vi "Process Mouse Up.vi"(0 "FSM.Graph in":T2, 5 "Display State In":T3, 7 "Coords":T4, 9 "PlatMods":T1, 11 "Editor Ref":refnum<vi>) -> (4 "FSM.Graph out":T2, 6 "Display State Out":T3, 10 "Refresh":bool)   [LabVIEW 2015, in "FSM Editor.xctl"]
uses:
  FSM Editor.xctl
  <vilib>/Utility/miscctls.llb/LVPoint32TypeDef.ctl
  State.vi
  Classes/FSM.Port/FSM.Port.lvclass
  Drag Mode.ctl
  Events.ctl
  NodeAdded.ctl
  NodeSelected.ctl
  EdgeEventData.ctl
  Data.vi
  Classes/FSM.Graph/FSM.Graph.lvclass
  Classes/FSM.Port/FSM.Port.lvclass/FSM.Port.ctl
  Classes/FSM.Graph/FSM.Graph.lvclass/FSM.Graph.ctl
  Classes/FSM.Port/Read belongsTo.vi
  Classes/FSM.Graph/Read selectedNodes.vi
  Classes/FSM.Graph/Read selectedEdge.vi
  Classes/FSM.Graph/Write selectedEdge.vi
  <vilib>/Utility/cursorutil.llb/Set Cursor (Icon Pict).vi
  Classes/FSM.Edge/FSM.Edge.lvclass
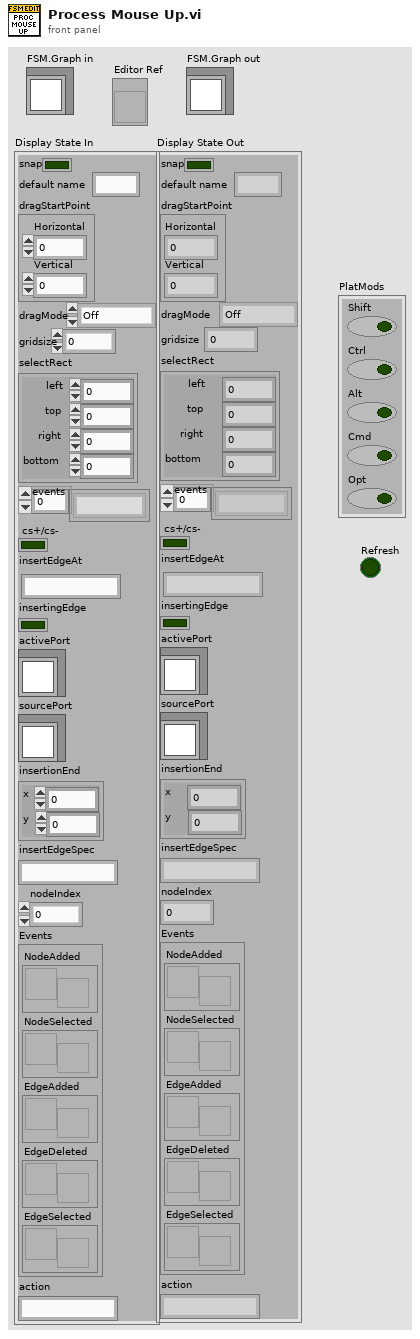
[diagram p1: front panel]
types:
  T1 = cluster{"Shift":bool, "Ctrl":bool, "Alt":bool, "Cmd":bool, "Opt":bool}
  T2 = typedef "FSM Editor.xctl/Data.vi" = refnum<class "FSM.Graph.lvclass">
  T3 = typedef "FSM Editor.xctl/State.vi" = cluster{"snap":bool, "default name":string, "dragStartPoint":T4, "dragMode":T5, "gridsize":dbl, "selectRect":cluster{"left":i16, "top":i16, "right":i16, "bottom":i16}, "events":string[], "cs+/cs-":bool, "insertEdgeAt":string, "insertingEdge":bool, "activePort":refnum<class "FSM.Port.lvclass">, "sourcePort":refnum<class "FSM.Port.lvclass">, "insertionEnd":cluster{"x":i16, "y":i16}, "insertEdgeSpec":string, "nodeIndex":i32, "Events":T6, "action":string}
  T4 = typedef "LVPoint32TypeDef.ctl" = cluster{"Horizontal":i32, "Vertical":i32}
  T5 = typedef "Drag Mode.ctl" = enum16{"Off", "NodePending", "Nodes", "Pan", "Select", "EdgeInsertion", "EdgePoint", "EdgeLabel"}
  T6 = typedef "FSM Editor.xctl/Events.ctl" = cluster{"NodeAdded":refnum<user-event>, "NodeSelected":refnum<user-event>, "EdgeAdded":refnum<user-event>, "EdgeDeleted":refnum<user-event>, "EdgeSelected":refnum<user-event>}
  T7 = enum16{"Off", "NodePending", "Nodes", "Pan", "Select", "EdgeInsertion", "EdgePoint", "Edgelabel"}
  T8 = cluster{"SourceName":string, "TargetName":string, "Accessors:Text":string, "Type":string}
  T9 = cluster{"left":i16, "top":i16, "right":i16, "bottom":i16}
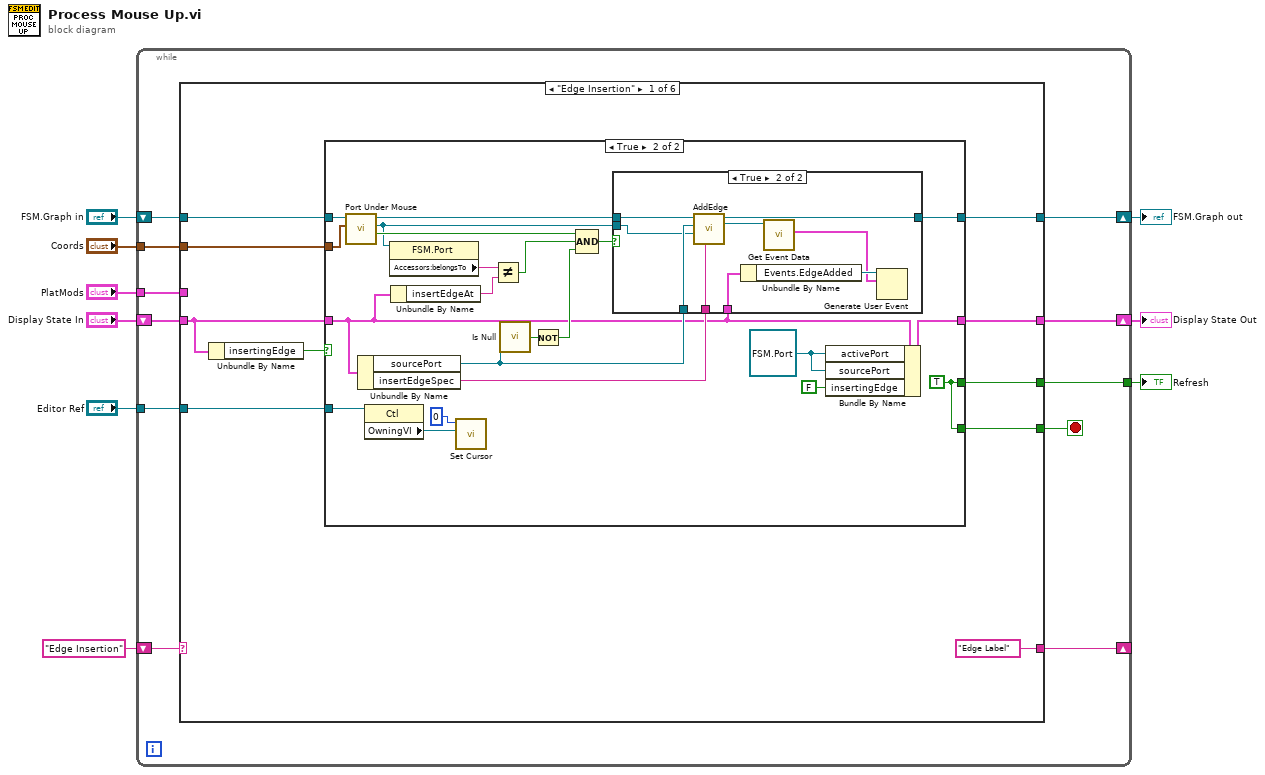
[diagram p0: block diagram]
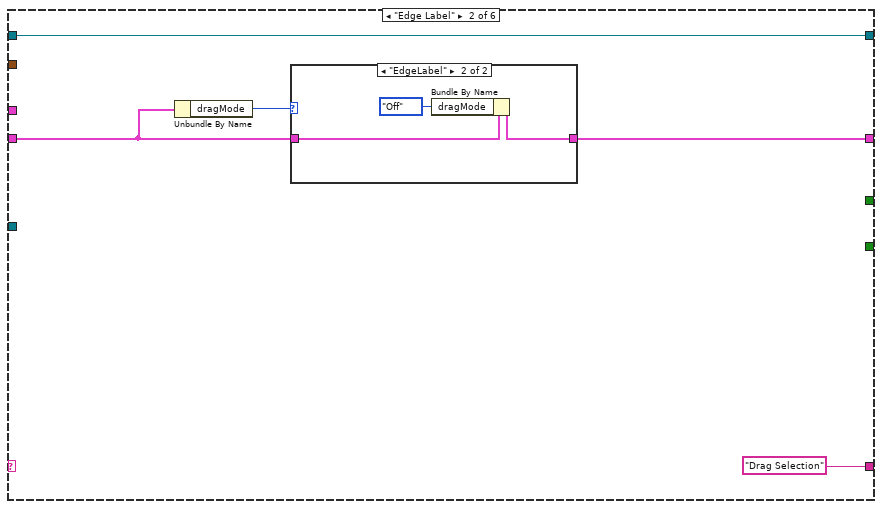
[diagram p4: hidden frame]
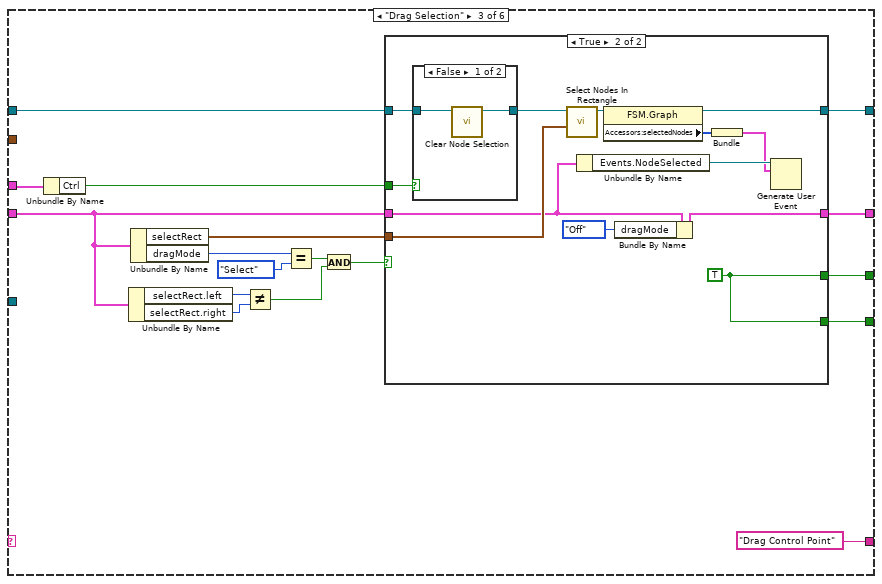
[diagram p6: hidden frame]
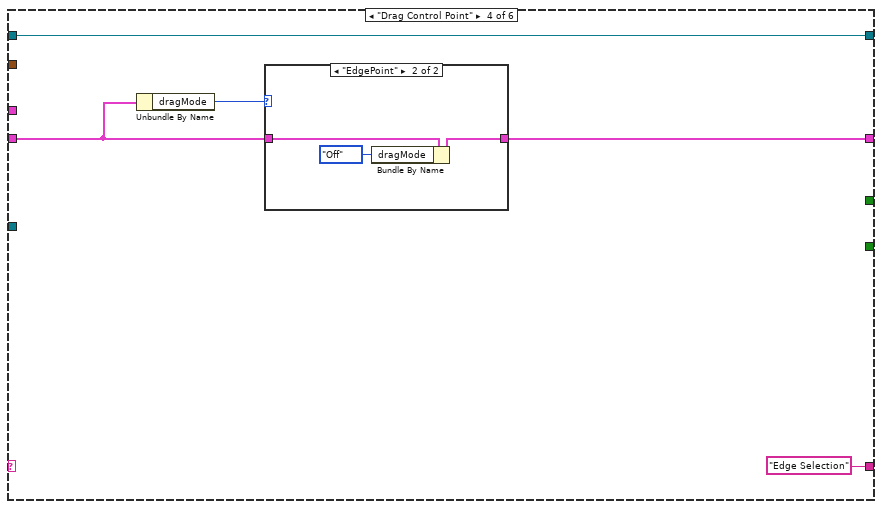
[diagram p9: hidden frame]
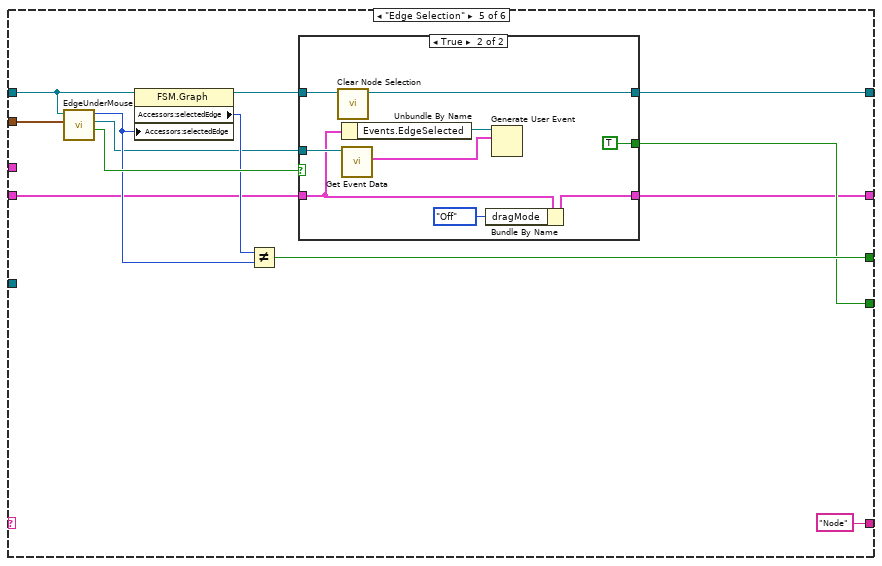
[diagram p11: hidden frame]
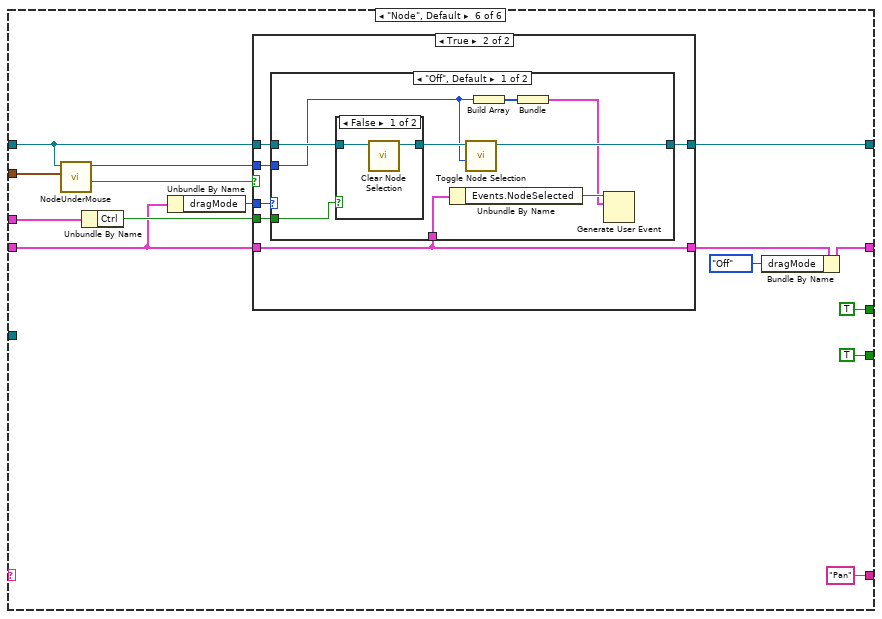
[diagram p13: hidden frame]
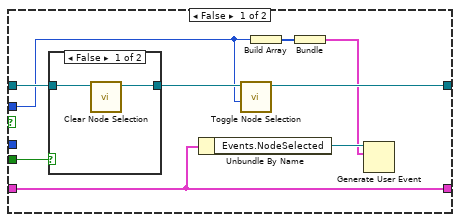
[diagram p14: hidden frame]
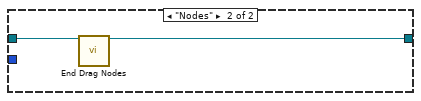
[diagram p17: hidden frame]
diagram:
  n1 = while {
    shift-right: [w18] -> w8
    shift-left: "FSM.Graph in" -> [w17]
    shift-right: [w19] -> _
    shift-left: "Edge Insertion" -> [w20]
    tunnel: "Coords" -> [w15]
    shift-right: [w14] -> w5
    shift-left: "Display State In" -> [w16]
    tunnel: [w12] -> w4
    tunnel: "PlatMods" -> [w11]
    tunnel: "Editor Ref" -> [w10]
    stop <- w13 stop-if-true
    n2 = case shown="\"Edge Insertion\"" w20 {
      tunnel: ["Edge Label" "Drag Selection" "Drag Control Point" "Edge Selection" "Node" "Pan"] -> w19
      tunnel: [w27 w68 w87 w112 w127 w155] -> w18
      tunnel: w17 -> [w28 w68 w88 w112 w122 w151]
      tunnel: w16 -> [w25 w66 w79 w110 w120 w145]
      tunnel: w15 -> [w21 _ _ _ w129 w150]
      tunnel: [w26 w67 w81 w109 w119 w152] -> w14
      tunnel: [w23 _ w85 _ w124 TRUE] -> w13
      tunnel: [w24 _ w86 _ w125 TRUE] -> w12
      tunnel: w11 -> [_ _ w84 _ _ w147]
      tunnel: w10 -> [w22 _ _ _ _ _]
      frame "Edge Insertion" {
        n3 = Unbundle By Name(w25) -> ("insertingEdge"=w29:bool)
        n4 = case shown="True" w29 {
          tunnel: w28 -> [w32 w53]
          tunnel: [w32 w39] -> w27
          tunnel: [w31 w47] -> w26
          tunnel: w25 -> [w31 w33]
          tunnel: [_ w54] -> w24
          tunnel: [_ w54] -> w23
          tunnel: w22 -> [_ w44]
          tunnel: w21 -> [_ w36]
          frame False {
          }
          frame True {
            w46 = refnum<class "FSM.Port.lvclass"> refnum ("activePort")
            w54 = TRUE
            n5 = call "Port Under Mouse.vi"("point"=w36, "FSM in"=w53) -> ("found?"=w52:bool, "Port"=w37:refnum<class "FSM.Port.lvclass">, "FSM out"=w41:T2)  [unwired: 6 in, 1 out]
            n6 = Unbundle By Name(w33) -> ("sourcePort"=w38:refnum<class "FSM.Port.lvclass">, "insertEdgeSpec"=w34:string)
            n7 = property class="Ctl"(reference=w44) -> ("OwningVI"=w43:refnum<vi>)  [unwired: 1 in, 2 out]
            n8 = property class="FSM.Port"(reference=w37) -> ("Accessors:belongsTo"=w49:string)  [unwired: 1 in, 2 out]
            n9 = Unbundle By Name(w33) -> ("insertEdgeAt"=w35:string)
            n10 = call-poly <vilib>:"Set Cursor.vi"("VI reference (current VI)"=w43, "icon"=u16 0) -> ()  [unwired: 8 in, 2 out]
            n11 = Not Equal?(x=w49, y=w35) -> (x != y?=w48:bool)
            n12 = call "Is Null.vi"("Port"=w38) -> ("null"=w51:bool)
            n13 = Not(x=w51) -> (.not. x?=w50:bool)
            n14 = Compound Arithmetic op=AND(w52, w48, w50) -> (w40:bool)
            n15 = case shown="True" w40 {
              tunnel: w41 -> [w55 w64]
              tunnel: [w55 w63] -> w39
              tunnel: w38 -> [_ w62]
              tunnel: w37 -> [_ w61]
              tunnel: w34 -> [_ w60]
              tunnel: w33 -> [_ w59]
              frame False {
              }
              frame True {
                n16 = call "AddEdge.vi"("edgeSpec"=w60, "Target Port"=w61, "Source Port"=w62, "FSM in"=w64) -> ("New Edge"=w57:refnum<class "FSM.Edge.lvclass">, "FSM out"=w63:T2)  [unwired: 5 in, 1 out]
                n17 = Unbundle By Name(w59) -> ("Events.EdgeAdded"=w58:refnum<user-event>)
                n18 = call "Get Event Data.vi"("FSM.Edge in"=w57) -> ("Event Data"=w56:T8)  [unwired: 8 in, 2 out]
                n19 = Generate User Event(user event=w58, event data cluster=w56) -> ()  [unwired: 2 in, 2 out]
              }
            }
            n20 = Bundle By Name(cluster=w33, "activePort"=w46, "sourcePort"=w46, "insertingEdge"=FALSE) -> (w47:T3)
          }
        }
      }
      frame "Edge Label" {
        n21 = Unbundle By Name(w66) -> ("dragMode"=w65:T5)
        n22 = case shown="\"EdgeLabel\"" w65 {
          tunnel: [w70 w73] -> w67
          tunnel: w66 -> [w70 w71]
          frame "Off", Default {
          }
          frame "EdgeLabel" {
            n23 = Bundle By Name(cluster=w71, "dragMode"=Drag_Mode."Off") -> (w73:T3)
          }
        }
      }
      frame "Drag Selection" {
        n24 = Unbundle By Name(w84) -> ("Ctrl"=w83:bool)
        n25 = Unbundle By Name(w79) -> ("selectRect.left"=w77:i16, "selectRect.right"=w78:i16)
        n26 = Unbundle By Name(w79) -> ("selectRect"=w82:T9, "dragMode"=w89:T5)
        n27 = Not Equal?(x=w77, y=w78) -> (x != y?=w75:bool)
        n28 = Equal?(x=w89, y=T7."Select") -> (x = y?=w76:bool)
        n29 = And(x=w76, y=w75) -> (x .and. y?=w74:bool)
        n30 = case shown="True" w74 {
          tunnel: w88 -> [w92 w103]
          tunnel: [w92 w95] -> w87
          tunnel: w79 -> [w91 w96]
          tunnel: [_ w105] -> w86
          tunnel: [_ w105] -> w85
          tunnel: w83 -> [_ w104]
          tunnel: w82 -> [_ w100]
          tunnel: [w91 w99] -> w81
          frame False {
          }
          frame True {
            w105 = TRUE
            n31 = case shown="False" w104 {
              tunnel: [w106 w108] -> w102
              tunnel: w103 -> [w107 w108]
              frame False {
                n32 = call "Clear Node Selection.vi"("FSM in"=w107) -> ("FSM out"=w106:T2)  [unwired: 9 in, 1 out]
              }
              frame True {
              }
            }
            n33 = call "Select Nodes In Rectangle.vi"("selectRect"=w100, "FSM in"=w102) -> ("FSM out"=w101:T2)  [unwired: 8 in, 1 out]
            n34 = Unbundle By Name(w96) -> ("Events.NodeSelected"=w97:refnum<user-event>)
            n35 = property class="FSM.Graph"(reference=w101) -> (reference out=w95:T2, "Accessors:selectedNodes"=w94:i32[])  [unwired: 1 in, 1 out]
            n36 = Bundle By Name(cluster=w96, "dragMode"=Drag_Mode."Off") -> (w99:T3)
            n37 = Bundle("Accessors:selectedNodes"=w94) -> (w93:cluster{"Accessors:selectedNodes":i32[]})  [unwired: 1 in]
            n38 = Generate User Event(user event=w97, event data cluster=w93) -> ()  [unwired: 2 in, 2 out]
          }
        }
      }
      frame "Drag Control Point" {
        n39 = Unbundle By Name(w110) -> ("dragMode"=w111:T5)
        n40 = case shown="\"EdgePoint\"" w111 {
          tunnel: w110 -> [w114 w117]
          tunnel: [w114 w116] -> w109
          frame "Off", Default {
          }
          frame "EdgePoint" {
            n41 = Bundle By Name(cluster=w117, "dragMode"=Drag_Mode."Off") -> (w116:T3)
          }
        }
      }
      frame "Edge Selection" {
        n42 = call "EdgeUnderMouse.vi"("Coords"=w129, "FSM in"=w122) -> ("contains mouse"=w128:bool, "Edge"=w118:refnum<class "FSM.Edge.lvclass">, "Edge Index"=w123:i32)  [unwired: 6 in, 1 out]
        n43 = property class="FSM.Graph"(reference=w122, "Accessors:selectedEdge"=w123) -> (reference out=w121:T2, "Accessors:selectedEdge"=w126:i32)  [unwired: 1 in, 1 out]
        n44 = Not Equal?(x=w126, y=w123) -> (x != y?=w125:bool)
        n45 = case shown="True" w128 {
          tunnel: w121 -> [w132 w141]
          tunnel: [w132 w140] -> w127
          tunnel: [_ TRUE] -> w124
          tunnel: w120 -> [w131 w135]
          tunnel: [w131 w138] -> w119
          tunnel: w118 -> [_ w136]
          frame False {
          }
          frame True {
            n46 = call "Clear Node Selection.vi"("FSM in"=w141) -> ("FSM out"=w140:T2)  [unwired: 9 in, 1 out]
            n47 = Unbundle By Name(w135) -> ("Events.EdgeSelected"=w134:refnum<user-event>)
            n48 = call "Get Event Data.vi"("FSM.Edge in"=w136) -> ("Event Data"=w133:T8)  [unwired: 8 in, 2 out]
            n49 = Bundle By Name(cluster=w135, "dragMode"=Drag_Mode."Off") -> (w138:T3)
            n50 = Generate User Event(user event=w134, event data cluster=w133) -> ()  [unwired: 2 in, 2 out]
          }
        }
      }
      frame "Node", Default {
        n51 = call "NodeUnderMouse.vi"("Coords"=w150, "FSM in"=w151) -> ("contains mouse"=w148:bool, "Node Index"=w143:i32)  [unwired: 6 in, 2 out]
        n52 = Unbundle By Name(w147) -> ("Ctrl"=w146:bool)
        n53 = Unbundle By Name(w145) -> ("dragMode"=w144:T5)
        n54 = case shown="True" w148 {
          tunnel: w151 -> [w165 w173]
          tunnel: [w162 w172] -> w155
          tunnel: [w161 w169] -> w154
          tunnel: w145 -> [w161 w169]
          tunnel: w146 -> [w164 w171]
          tunnel: w144 -> [_ w174]
          tunnel: w143 -> [w159 w170]
          frame False {
            n55 = case shown="False" w164 {
              tunnel: w165 -> [w167 w168]
              tunnel: [w166 w168] -> w163
              frame False {
                n56 = call "Clear Node Selection.vi"("FSM in"=w167) -> ("FSM out"=w166:T2)  [unwired: 9 in, 1 out]
              }
              frame True {
              }
            }
            n57 = Unbundle By Name(w161) -> ("Events.NodeSelected"=w160:refnum<user-event>)
            n58 = call "Toggle Node Selection.vi"("New selection"=w159, "FSM in"=w163) -> ("FSM out"=w162:T2)  [unwired: 8 in, 1 out]
            n59 = Build Array(w159) -> (w158:i32[])
            n60 = Bundle(w158) -> (w157:cluster{i32[]})  [unwired: 1 in]
            n61 = Generate User Event(user event=w160, event data cluster=w157) -> ()  [unwired: 2 in, 2 out]
          }
          frame True {
            n62 = case shown="\"Off\", Default" w174 {
              tunnel: w173 -> [w183 w188]
              tunnel: [w180 w187] -> w172
              tunnel: w171 -> [w182 _]
              tunnel: w170 -> [w178 _]
              tunnel: w169 -> [w176 _]
              frame "Off", Default {
                n63 = case shown="False" w182 {
                  tunnel: w183 -> [w185 w186]
                  tunnel: [w184 w186] -> w181
                  frame False {
                    n64 = call "Clear Node Selection.vi"("FSM in"=w185) -> ("FSM out"=w184:T2)  [unwired: 9 in, 1 out]
                  }
                  frame True {
                  }
                }
                n65 = Unbundle By Name(w176) -> ("Events.NodeSelected"=w177:refnum<user-event>)
                n66 = call "Toggle Node Selection.vi"("New selection"=w178, "FSM in"=w181) -> ("FSM out"=w180:T2)  [unwired: 8 in, 1 out]
                n67 = Build Array(w178) -> (w179:i32[])
                n68 = Bundle(w179) -> (w175:cluster{i32[]})  [unwired: 1 in]
                n69 = Generate User Event(user event=w177, event data cluster=w175) -> ()  [unwired: 2 in, 2 out]
              }
              frame "Nodes" {
                n70 = call "End Drag Nodes.vi"("FSM in"=w188) -> ("FSM out"=w187:T2)  [unwired: 13 in, 1 out]
              }
            }
          }
        }
        n71 = Bundle By Name(cluster=w154, "dragMode"=Drag_Mode."Off") -> (w152:T3)
      }
    }
  }
  "Display State Out" <- w5
  "FSM.Graph out" <- w8
  "Refresh" <- w4
